vi "Inventory-CheckAdmin.vi"(8 "error in (no error)":errorcluster, 11 "Tab Control - Finished Goods":refnum<vi>) -> (0 "error out":errorcluster)   [LabVIEW 2013, in "ERP-Inventory.lvclass"]
uses:
  ERP-Inventory.lvclass
  Globals/Global-SystemSettings.vi
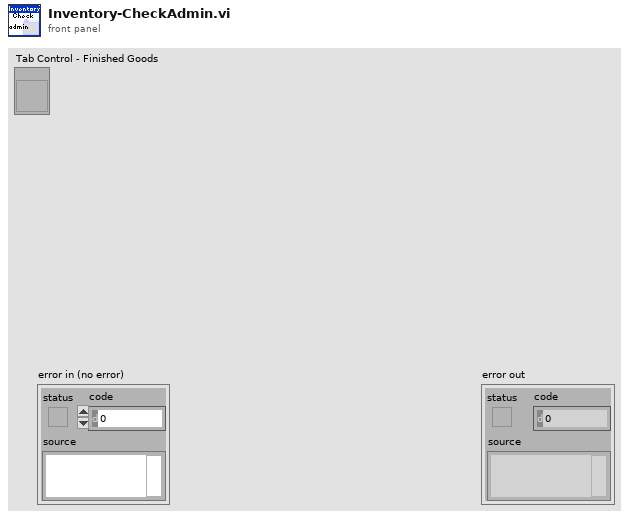
[diagram p1: front panel]
types:
  T1 = enum32{"Intro Page", "Finished Goods Inventory", "Raw Goods Inventory", "Admin"}
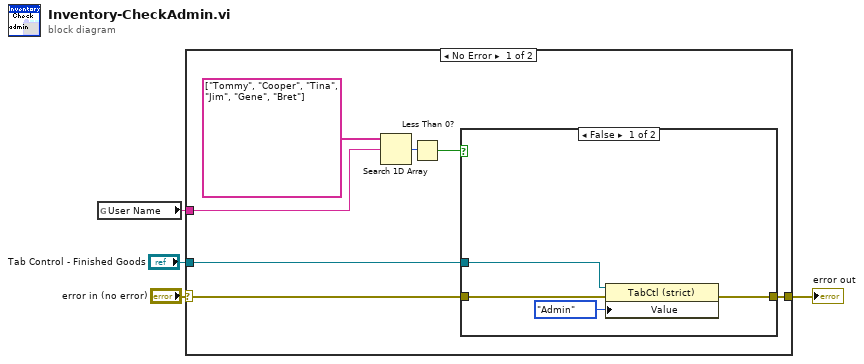
[diagram p0: block diagram]
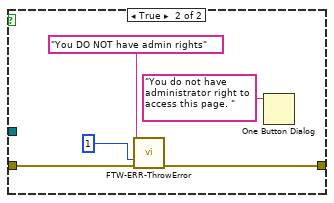
[diagram p2: hidden frame]
diagram:
  n1 = global read "Global-SystemSettings.vi" "User Name"() -> (w2:string)
  n2 = case shown="No Error" "error in (no error)" {
    selector: "error in (no error)" -> [w8 w21]
    tunnel: [w7 w21] -> w3
    tunnel: "Tab Control - Finished Goods" -> [w6 _]
    tunnel: w2 -> [w5 _]
    frame No Error {
      n3 = Search 1D Array(1D array=string[] ["Tommy", "Cooper", "Tina", "Jim", "Gene", "Bret"], element=w5) -> (index of element=w10:i32)  [unwired: 1 in]
      n4 = Less Than 0?(x=w10) -> (x < 0?=w9:bool)
      n5 = case shown="False" w9 {
        tunnel: w8 -> [w15 w20]
        tunnel: [w14 w17] -> w7
        tunnel: w6 -> [w13 _]
        frame False {
          n6 = property on="Property Node" class="TabCtl (strict)"(reference=w13, error in=w15, "Value"=T1."Admin") -> (error out=w14:errorcluster)  [unwired: 1 out]
        }
        frame True {
          n7 = call "FTW-ERR-ThrowError.vi"("Error Message"="You DO NOT have admin rights", "Error Code"=1, "error in"=w20) -> ("error out"=w17:errorcluster)  [unwired: 12 in]
          n8 = One Button Dialog(message="You do not have administrator right to access this page. ") -> ()  [unwired: 1 in, 1 out]
        }
      }
    }
    frame Error {
    }
  }
  "error out" <- w3
